vi "downsample.vi"(2 "error in":errorcluster, 3 "img dst":T1, 4 "downsampling":i32=24, 5 "img src":T1) -> (0 "error out":errorcluster, 1 "Image Dst Out":T1)   [LabVIEW 2012]
uses:
  <vilib>/vision/Image Controls.llb/IMAQ Image.ctl
  <resource>/objmgr/IMAQImage.rc
  <vilib>/vision/NI_Vision_Development_Module.lvlib
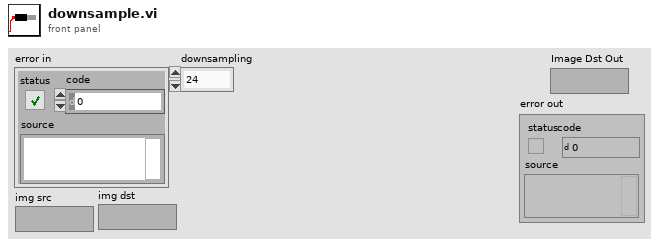
[diagram p1: front panel]
types:
  T1 = typedef "IMAQ Image.ctl" = refnum<image>
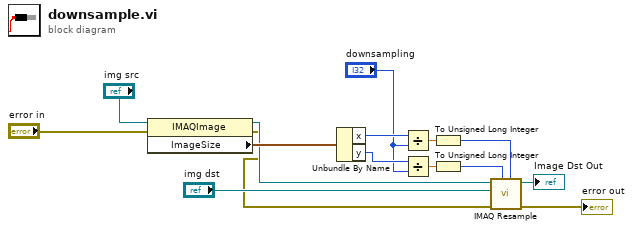
[diagram p0: block diagram]
diagram:
  n1 = property class="IMAQImage"(reference="img src", error in="error in") -> (reference out=w7:T1, error out=w1:errorcluster, "ImageSize"=w15:cluster{"x":i32, "y":i32})
  n2 = Unbundle By Name(w15) -> ("x"=w14:i32, "y"=w13:i32)
  n3 = Divide(x=w14, y="downsampling") -> (x/y=w11:dbl)
  n4 = Divide(x=w13, y="downsampling") -> (x/y=w10:dbl)
  n5 = To Unsigned Long Integer(number=w11) -> (unsigned 32bit integer=w9:u32)
  n6 = To Unsigned Long Integer(number=w10) -> (unsigned 32bit integer=w8:u32)
  n7 = call "IMAQ Resample"("X Resolution"=w9, "Y Resolution"=w8, "error in (no error)"=w1, "Image Dst"="img dst", "Image Src"=w7) -> ("error out"=→"error out":errorcluster, "Image Dst Out"=→"Image Dst Out":T1)  [unwired: 5 in]
